vi "PM-control_waveform_size.vi"(7 "Clear waveform":bool, 9 "Samples s":i32, 10 "old waveform":waveform(dbl), 11 "New waveform":waveform(dbl)) -> (2 "waveform":waveform(dbl))   [LabVIEW 2018]
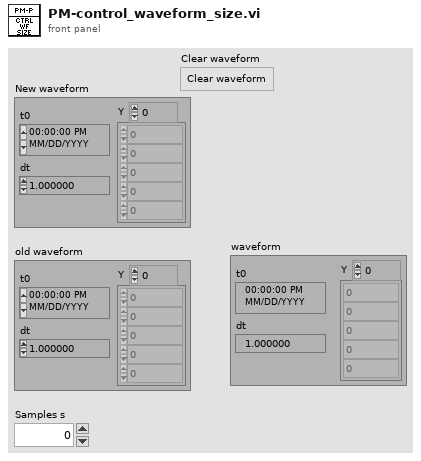
[diagram p1: front panel]
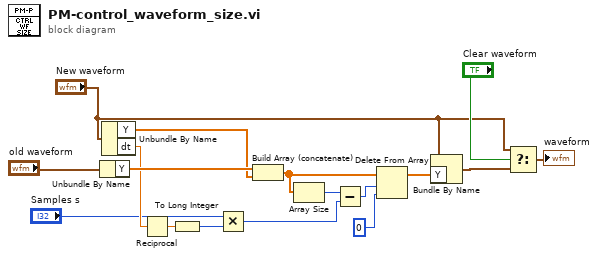
[diagram p0: block diagram]
diagram:
  n1 = Unbundle By Name("old waveform") -> ("Y"=w16:dbl[])
  n2 = Unbundle By Name("New waveform") -> ("Y"=w10:dbl[], "dt"=w11:dbl)
  n3 = Reciprocal(x=w11) -> (1/x=w12:dbl)
  n4 = To Long Integer(number=w12) -> (32bit integer=w7:i32)
  n5 = Multiply(x="Samples s", y=w7) -> (x*y=w5:i32)
  n6 = Build Array (concatenate)(w16, w10) -> (w8:dbl[])
  n7 = Array Size(array=w8) -> (size(s)=w9:i32)
  n8 = Subtract(x=w9, y=w5) -> (x-y=w13:i32)
  n9 = Delete From Array(array=w8, length=w13, index=0) -> (array with subset deleted=w17:dbl[])  [unwired: 1 out]
  n10 = Bundle By Name(cluster="New waveform", "Y"=w17) -> (w3:waveform(dbl))
  n11 = Select(t="New waveform", s="Clear waveform", f=w3) -> (s? t:f=→"waveform":waveform(dbl))
